vi "Write NumberOfTactics.vi"(8 "error in (no error)":errorcluster, 10 "NumberOfTactics":dbl=3.0, 11 "ABCThirdKicker in":refnum<class "ABCThirdKicker.lvclass">) -> (0 "error out":errorcluster, 3 "ABCThirdKicker out":refnum<class "ABCThirdKicker.lvclass">)   [LabVIEW 2020, in "ABCThirdKicker.lvclass"]
uses:
  ABCThirdKicker.lvclass
  ABCThirdKicker.lvclass/ABCThirdKicker.ctl
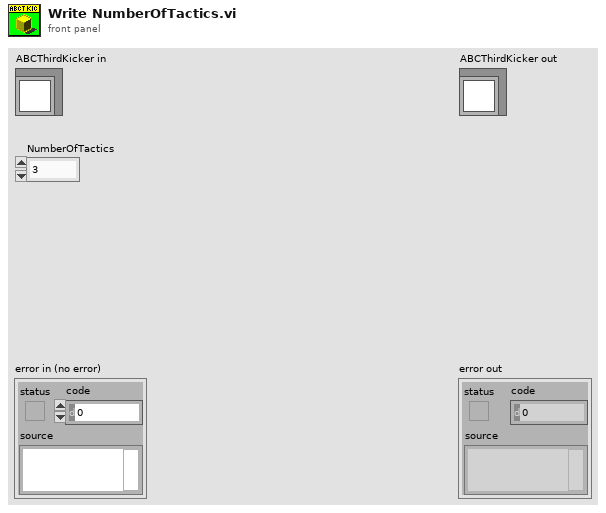
[diagram p1: front panel]
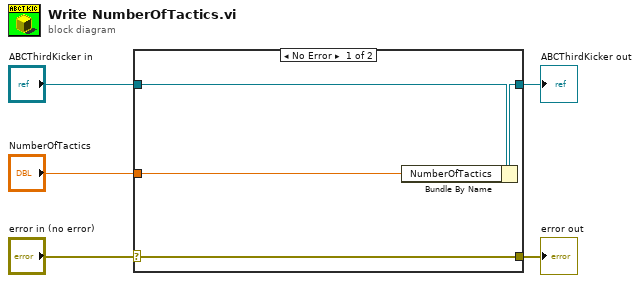
[diagram p0: block diagram]
diagram:
  n1 = case shown="No Error" "error in (no error)" {
    selector: "error in (no error)" -> [w9 w10]
    tunnel: [w9 w10] -> w4
    tunnel: [w7 w11] -> w2
    tunnel: "ABCThirdKicker in" -> [w8 w11]
    tunnel: "NumberOfTactics" -> [w6 _]
    frame No Error {
      n2 = Bundle By Name(cluster=w8, "NumberOfTactics"=w6) -> (w7:refnum<class "ABCThirdKicker.lvclass">)
    }
    frame Error {
    }
  }
  "error out" <- w4
  "ABCThirdKicker out" <- w2
